vi "ohm_law.vi"() -> ()   [LabVIEW 2023]
uses:
  <vilib>/Analysis/NI_AALPro.lvlib
  <vilib>/Analysis/6fits.llb/Confidence Interval (Linear).vi
  <vilib>/Utility/file.llb/Write Delimited Spreadsheet (DBL).vi
panel:
  in  "Esci":bool
  in  "Salva dati":bool
  out "Fit I-V":cluster{dbl[], "Best Linear Fit":dbl[]}[](graph)
  out "R (Ohm)":dbl
  out "delta R (Ohm)":dbl
  out "delta m":dbl
  out "delta q":dbl
  out "m":dbl
  out "q":dbl
  in  "Analizza I-V":bool caption="OK Button"
  out "I-V":cluster{dbl[], dbl[]}(graph)
  in  "Misura I-V":bool caption="OK Button"
  in  "N divisioni":i32
  in  "Vmin":dbl min=-5.0 max=0.0 step=1.0
  in  "Vmax":dbl min=0.0 max=5.0 step=1.0
  in  "Device Name":tag
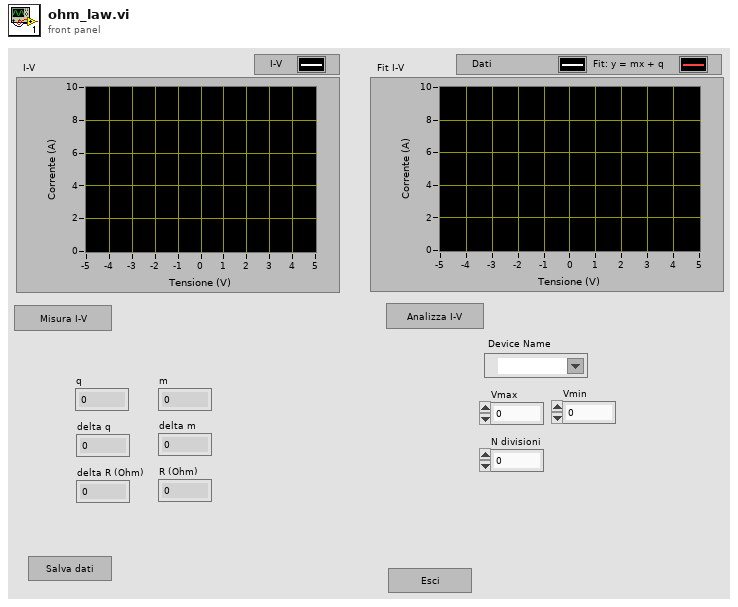
[diagram p1: front panel]
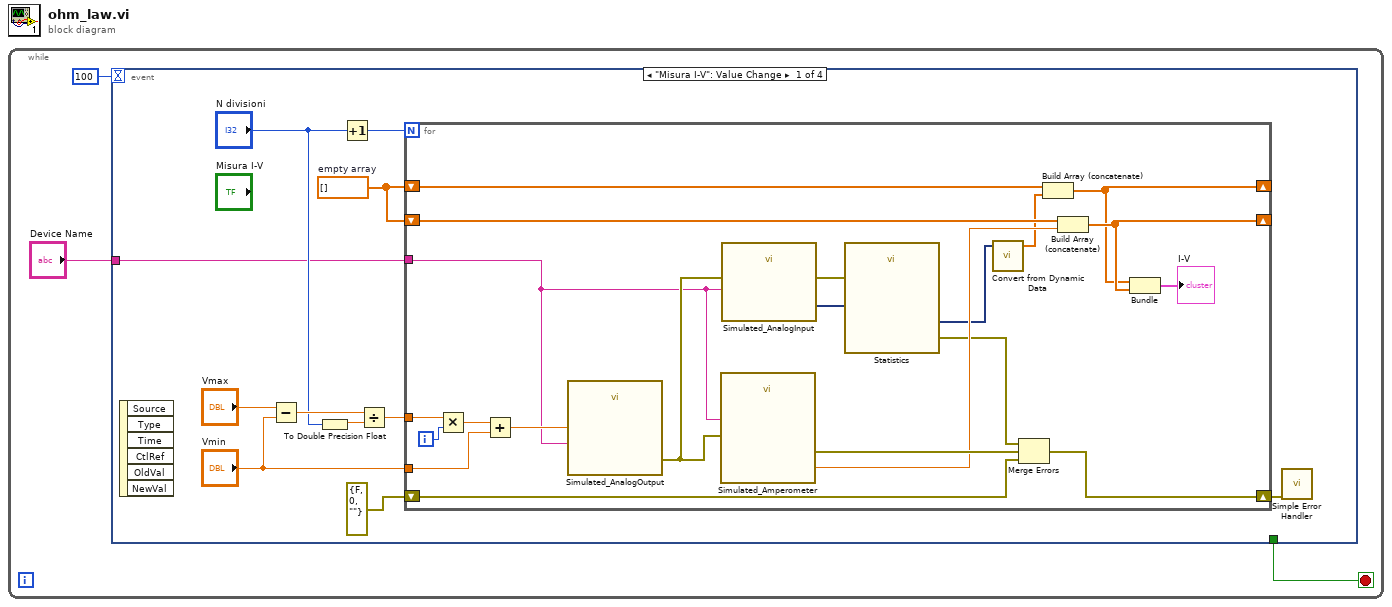
[diagram p0: block diagram]
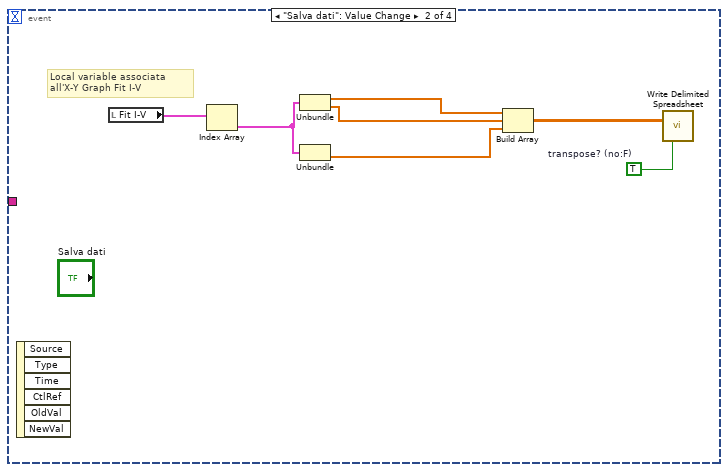
[diagram p2: hidden frame]
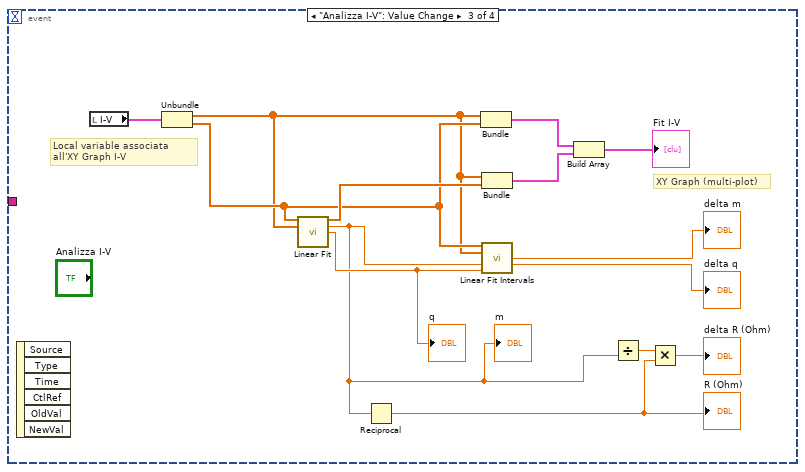
[diagram p3: hidden frame]
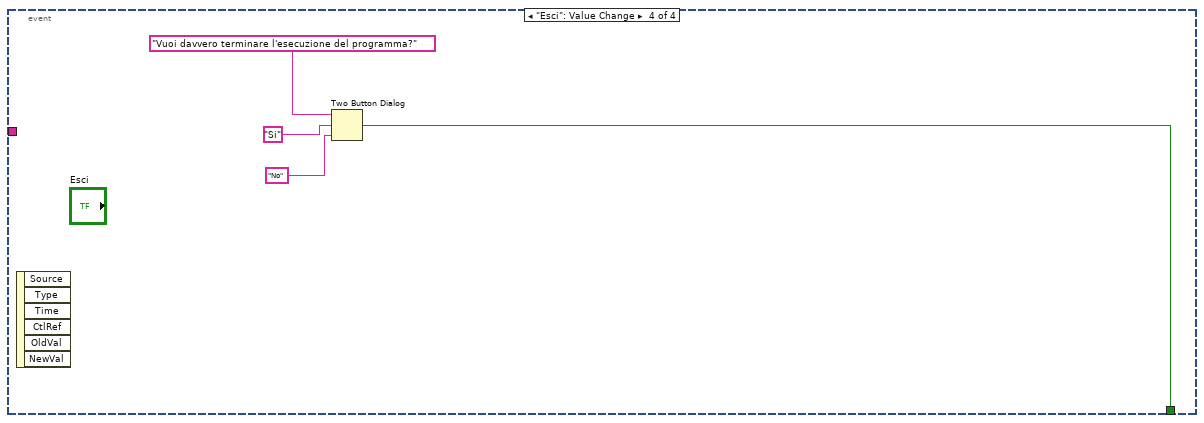
[diagram p4: hidden frame]
diagram:
  n1 = while {
    stop <- w1 stop-if-true
    n2 = event shown="[0] \"Misura I-V\": Value Change" {
      selector: _ -> [_ _ _ _]
      dyn-events: _ -> [_ _ _ _]
      timeout: 100 -> [_ _ _ _]
      tunnel: "Device Name" -> [w7 _ _ _]
      tunnel: [_ _ _ w57] -> w1
      event "Misura I-V": Value Change {
        w6 = dbl[] []  # empty array
        n3 = event-data() -> ()  [unwired: 1 in, 6 out]
        n4 = Subtract(x="Vmax", y="Vmin") -> (x-y=w14:dbl)
        n5 = To Double Precision Float(number="N divisioni") -> (double precision float=w12:dbl)
        n6 = Increment(x="N divisioni") -> (x+1=w10:i32)
        n7 = Divide(x=w14, y=w12) -> (x/y=w9:dbl)
        n8 = for {
          N: w10 -> [_]
          tunnel: w9 -> [w34]
          tunnel: "Vmin" -> [w32]
          tunnel: w7 -> [w20]
          shift-right: [w24] -> _
          shift-left: w6 -> [w29]
          shift-right: [w23] -> _
          shift-left: w6 -> [w30]
          shift-right: [w21] -> w4
          shift-left: errorcluster {"status"=FALSE, "code"=0, "source"=""} ("error out") -> [w22]
          i -> [w35]
          n9 = Multiply(x=w34, y=w35) -> (x*y=w33:dbl)
          n10 = Add(x=w33, y=w32) -> (x+y=w31:dbl)
          n11 = call "Simulated_AnalogOutput.vi"("data"=w31, "Device Name"=w20) -> ("error out"=w28:errorcluster)  [unwired: 9 in]
          n12 = call "Simulated_Amperometer.vi"("error in (no error)"=w28, "Device Name"=w20) -> ("error out"=w27:errorcluster, "Measurement"=w26:dbl)  [unwired: 8 in]
          n13 = call "Simulated_AnalogInput.vi"("error in (no error)"=w28, "Device Name"=w20) -> ("error out"=w15:errorcluster, "data"=w18:dynamicdata)  [unwired: 8 in]
          n14 = call "Statistics"("Signals"=w18, "error in (no error)"=w15) -> ("Arithmetic Mean"=w16:dynamicdata, "error out"=w17:errorcluster)  [unwired: 24 in]
          n15 = call "Convert from Dynamic Data"("Dynamic Data Type"=w16) -> ("Array"=w19:dbl[])  [unwired: 3 in]
          n16 = Merge Errors "Merge Errors"(w17, w27, w22) -> (w21:errorcluster)
          n17 = Build Array (concatenate) "Build Array"(w30, w19) -> (w23:dbl[])
          n18 = Build Array (concatenate)(w29, w26) -> (w24:dbl[])
          n19 = Bundle "Bundle"(w23, w24) -> (→"I-V":cluster{dbl[], dbl[]})  [unwired: 1 in]
        }
        n20 = call <vilib>:"Simple Error Handler.vi"("error in (no error)"=w4) -> ()  [unwired: 4 in, 5 out]
      }
      event "Salva dati": Value Change {
        w36 = TRUE  # transpose? (no:F)
        # "Local variable associata all'X-Y Graph Fit I-V"
        n21 = event-data() -> ()  [unwired: 1 in, 6 out]
        n22 = local read "Fit I-V"() -> (w42:cluster{dbl[], "Best Linear Fit":dbl[]}[])
        n23 = Index Array(array=w42) -> (element=w41:cluster{dbl[], "Best Linear Fit":dbl[]})  [unwired: 1 in]
        n24 = Unbundle(w41) -> (w38:dbl[], "Best Linear Fit"=w39:dbl[])
        n25 = Unbundle(w41) -> ("Best Linear Fit"=w40:dbl[])  [unwired: 1 out]
        n26 = Build Array(w38, w39, w40) -> (w37:dbl[][])
        n27 = call-poly <vilib>:"Write Delimited Spreadsheet.vi"("2D data"=w37, "transpose? (no:F)"=w36) -> ()  [unwired: 12 in, 2 out]
      }
      event "Analizza I-V": Value Change {
        # "Local variable associata all'XY Graph I-V"
        # "XY Graph (multi-plot)"
        n28 = event-data() -> ()  [unwired: 1 in, 6 out]
        n29 = local read "I-V"() -> (w56:cluster{dbl[], dbl[]})
        n30 = Unbundle "Unbundle"(w56) -> (w53:dbl[], w54:dbl[])
        n31 = call <vilib>:"Linear Fit.vi"("Y"=w54, "X"=w53) -> ("Best Linear Fit"=w55:dbl[], "slope"=w51:dbl, "intercept"=w52:dbl)  [unwired: 9 in, 2 out]
        "q" <- w52
        "m" <- w51
        n32 = Reciprocal(x=w51) -> (1/x=w48:dbl)
        "R (Ohm)" <- w48
        n33 = Bundle(w53, w54) -> (w45:cluster{dbl[], dbl[]})  [unwired: 1 in]
        n34 = Bundle(w53, "Best Linear Fit"=w55) -> (w44:cluster{dbl[], "Best Linear Fit":dbl[]})  [unwired: 1 in]
        n35 = call-poly <vilib>:"Linear Fit Intervals.vi"("Y"=w54, "X"=w53, "slope"=w51, "intercept"=w52) -> ("delta slope"=→"delta m":dbl, "delta intercept"=→"delta q":dbl)  [unwired: 7 in, 3 out]
        n36 = Build Array(w45, w44) -> (→"Fit I-V":cluster{dbl[], "Best Linear Fit":dbl[]}[])
        n37 = Divide(y=w51) -> (x/y=w50:dbl)  [unwired: 1 in]
        n38 = Multiply(x=w50, y=w48) -> (x*y=→"delta R (Ohm)":dbl)
      }
      event "Esci": Value Change {
        n39 = event-data() -> ()  [unwired: 1 in, 6 out]
        n40 = Two Button Dialog(message="Vuoi davvero terminare l'esecuzione del programma?", 1:"No", 2:"Si") -> (T button?=w57:bool)
      }
    }
  }
